vi "HEWH Build String Diagnostics Data.vi"(1 "GEA2":bool, 2 "Pilot (SCFH)":dbl, 5 "ERD Data  2":T6, 9 "ERD Data":string[][](array[string]), 11 "Error In":errorcluster, 12 "Get Gas Data":bool, 13 "Measurement Data":T5, 14 "HEWH Specific DAQ":T1={"HEWH Data"={"HEWH Standard"={"Voltage (Volts)"=-1.0, "Current (Amps)"=-1.0, "Power (Watts)"=-1.0, "WattHours (Wh)"=-1.0, "TC Tree (AVG)"=0.0, "Flow Rate (GPM)"=0.0, "Gallons (Gal)"=0.0, "RTD Out (Deg F)"=0.0, "RTD In (Deg F)"=0.0, "RTD Amb (Deg F)"=0.0, "TC Down"=0.0, "UE Event Lead"=0, "LE Event Lead"=0, "TC Tree Array"=[]}, "PRAT"={"Power (Watts) A"=0.0, "Power (Watts) B"=0.0, "Power (Watts) C"=0.0, "Power (Watts) D"=0.0, "TC1"=0.0, "TC2"=0.0, "TC3"=0.0, "TC4"=0.0, "WattHours (Wh) A"=0.0, "WattHours (Wh) B"=0.0, "WattHours (Wh) C"=0.0, "WattHours (Wh) D"=0.0, "Ambient"=0.0, "Extra Temp"=0.0}, "Additional Power Data"={"Vthd"=0.0, "Frequency (Hz)"=0.0, "Apparent Power (VA)"=0.0, "Power Factor"=0.0, "Current Crest Factor"=0.0, "Voltage Crest Factor"=0.0, "Integration Time (sec)"=0.0}}, "Flow Valve % Open"=0.0, "Power State"={"UE"=FALSE, "LE"=FALSE, "COMP"=FALSE, "FANS"=FALSE}, "Power Analyzer"=enum."APLUS", "Flow Valve uA Output"=0, "Gallons Start (Gal)"=0.0, "PI Output"=0.0}) -> (6 "Power Display":T3, 10 "Appliance Data":string[][](array[string]), 15 "Error Out":errorcluster)   [LabVIEW 2020]
uses:
  Type Definitions/HEWH Power Elements.ctl
  Drivers/GEA3 Toolkit/LabVIEW GEA3 Rev2 API Toolkit LV2016/Water Heating Specific/Type Definitions/GEA3 HEWH ERD Data.ctl
  Drivers/GEA3 Toolkit/LabVIEW GEA3 Rev2 API Toolkit LV2016/Water Heating Specific/Type Definitions/GEA3 HEWH Mixing Valve.ctl
  Drivers/Alicat Gas Meter Driver/Sub-VIs/Data Cluster.ctl
  Type Definitions/HEWH Specific DAQ.ctl
  Type Definitions/HEWH Power Data.ctl
  Utility/Type Definitions/UTILITY Power Analyzer.ctl
panel:
  # "Totalizer Timer"
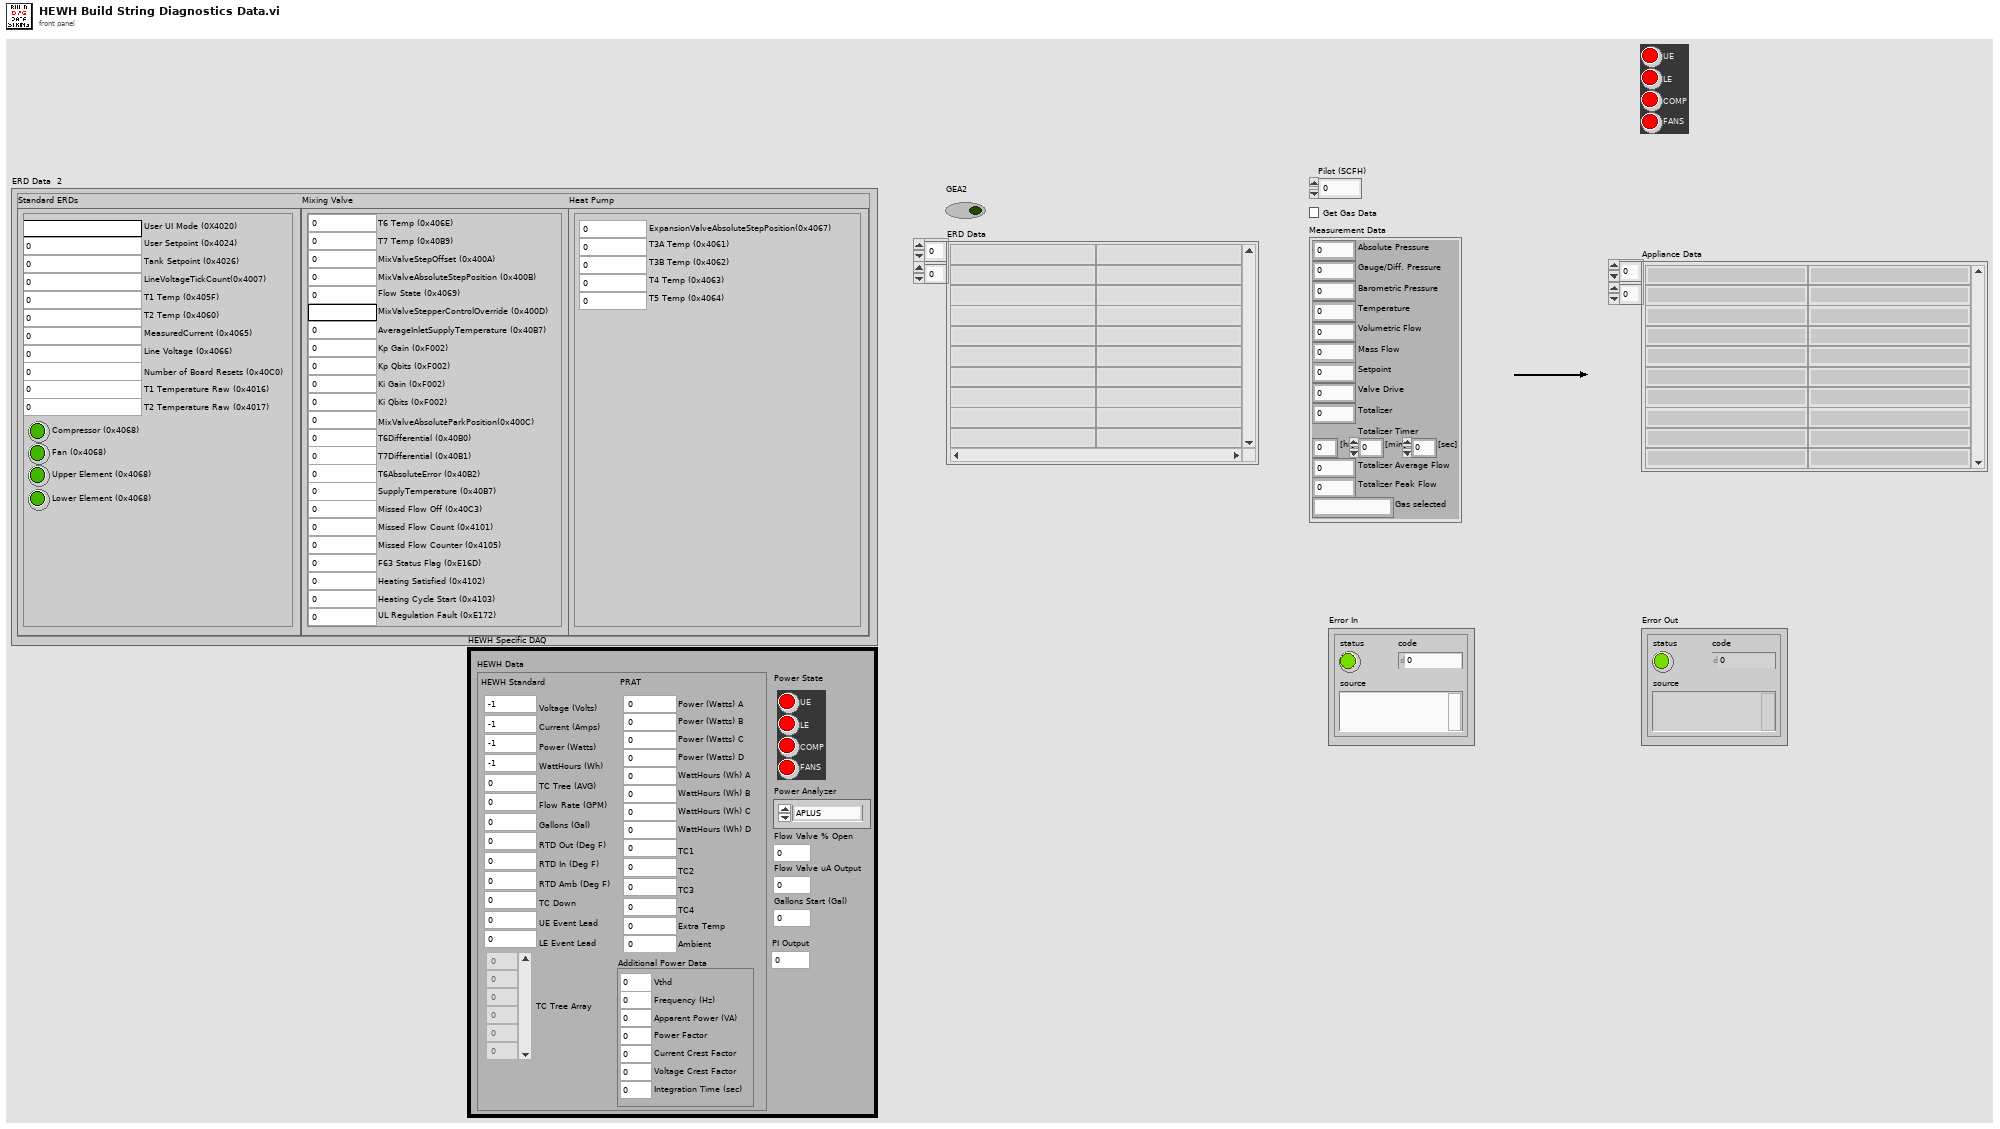
[diagram p1: front panel]
types:
  T1 = typedef "HEWH Specific DAQ.ctl" = cluster{"HEWH Data":T2, "Flow Valve % Open":dbl, "Power State":T3, "Power Analyzer":T4, "Flow Valve uA Output":i32, "Gallons Start (Gal)":dbl, "PI Output":dbl}
  T2 = typedef "HEWH Power Data.ctl" = cluster{"HEWH Standard":cluster{"Voltage (Volts)":dbl, "Current (Amps)":dbl, "Power (Watts)":dbl, "WattHours (Wh)":dbl, "TC Tree (AVG)":dbl, "Flow Rate (GPM)":dbl, "Gallons (Gal)":dbl, "RTD Out (Deg F)":dbl, "RTD In (Deg F)":dbl, "RTD Amb (Deg F)":dbl, "TC Down":dbl, "UE Event Lead":i32, "LE Event Lead":i32, "TC Tree Array":dbl[]}, "PRAT":cluster{"Power (Watts) A":dbl, "Power (Watts) B":dbl, "Power (Watts) C":dbl, "Power (Watts) D":dbl, "TC1":dbl, "TC2":dbl, "TC3":dbl, "TC4":dbl, "WattHours (Wh) A":dbl, "WattHours (Wh) B":dbl, "WattHours (Wh) C":dbl, "WattHours (Wh) D":dbl, "Ambient":dbl, "Extra Temp":dbl}, "Additional Power Data":cluster{"Vthd":dbl, "Frequency (Hz)":dbl, "Apparent Power (VA)":dbl, "Power Factor":dbl, "Current Crest Factor":dbl, "Voltage Crest Factor":dbl, "Integration Time (sec)":dbl}}
  T3 = typedef "HEWH Power Elements.ctl" = cluster{"UE":bool, "LE":bool, "COMP":bool, "FANS":bool}
  T4 = typedef "UTILITY Power Analyzer.ctl" = enum16{"", "APLUS", "WT210", "WT500", "WT300", "OSI", "Debug", "WT230", "WT300_1", "WT300_2"}
  T5 = typedef "Data Cluster.ctl" = cluster{"Absolute Pressure":dbl, "Gauge/Diff. Pressure":dbl, "Barometric Pressure":dbl, "Temperature":dbl, "Volumetric Flow":dbl, "Mass Flow":dbl, "Setpoint":dbl, "Valve Drive":dbl, "Totalizer":dbl, "[hr]":dbl, "[min]":dbl, "[sec]":dbl, "Totalizer Average Flow":dbl, "Totalizer Peak Flow":dbl, "Gas selected":string}
  T6 = typedef "GEA3 HEWH ERD Data.ctl" = cluster{"Mixing Valve":T7, "Standard ERDs":cluster{"User UI Mode (0X4020)":string, "User Setpoint (0x4024)":u16, "Compressor (0x4068)":bool, "Lower Element (0x4068)":bool, "Upper Element (0x4068)":bool, "Fan (0x4068)":bool, "T1 Temp (0x405F)":dbl, "T2 Temp (0x4060)":dbl, "Line Voltage (0x4066)":dbl, "MeasuredCurrent (0x4065)":dbl, "LineVoltageTickCount(0x4007)":u16, "Number of Board Resets (0x40C0)":u16, "T1 Temperature Raw (0x4016)":u16, "T2 Temperature Raw (0x4017)":u16, "Tank Setpoint (0x4026)":u16}, "Heat Pump":cluster{"ExpansionValveAbsoluteStepPosition(0x4067)":i16, "T3A Temp (0x4061)":dbl, "T3B Temp (0x4062)":dbl, "T4 Temp (0x4063)":dbl, "T5 Temp (0x4064)":dbl}}
  T7 = typedef "GEA3 HEWH Mixing Valve.ctl" = cluster{"T7 Temp (0x40B9)":dbl, "MixValveStepOffset (0x400A)":i16, "MixValveAbsoluteStepPosition (0x400B)":i16, "Flow State (0x4069)":u8, "MixValveStepperControlOverride (0x400D)":string, "AverageInletSupplyTemperature (0x40B7)":dbl, "T6 Temp (0x406E)":dbl, "Kp Gain (0xF002)":u16, "Kp Qbits (0xF002)":u16, "Ki Gain (0xF002)":u16, "Ki Qbits (0xF002)":u16, "MixValveAbsoluteParkPosition(0x400C)":i16, "T7Differential (0x40B1)":dbl, "T6Differential (0x40B0)":dbl, "SupplyTemperature (0x40B7)":dbl, "Missed Flow Off (0x40C3)":u8, "T6AbsoluteError (0x40B2)":dbl, "Missed Flow Count (0x4101)":u16, "Missed Flow Counter (0x4105)":u16, "F63 Status Flag (0xE16D)":u16, "Heating Satisfied (0x4102)":u16, "Heating Cycle Start (0x4103)":u16, "UL Regulation Fault (0xE172)":u8}
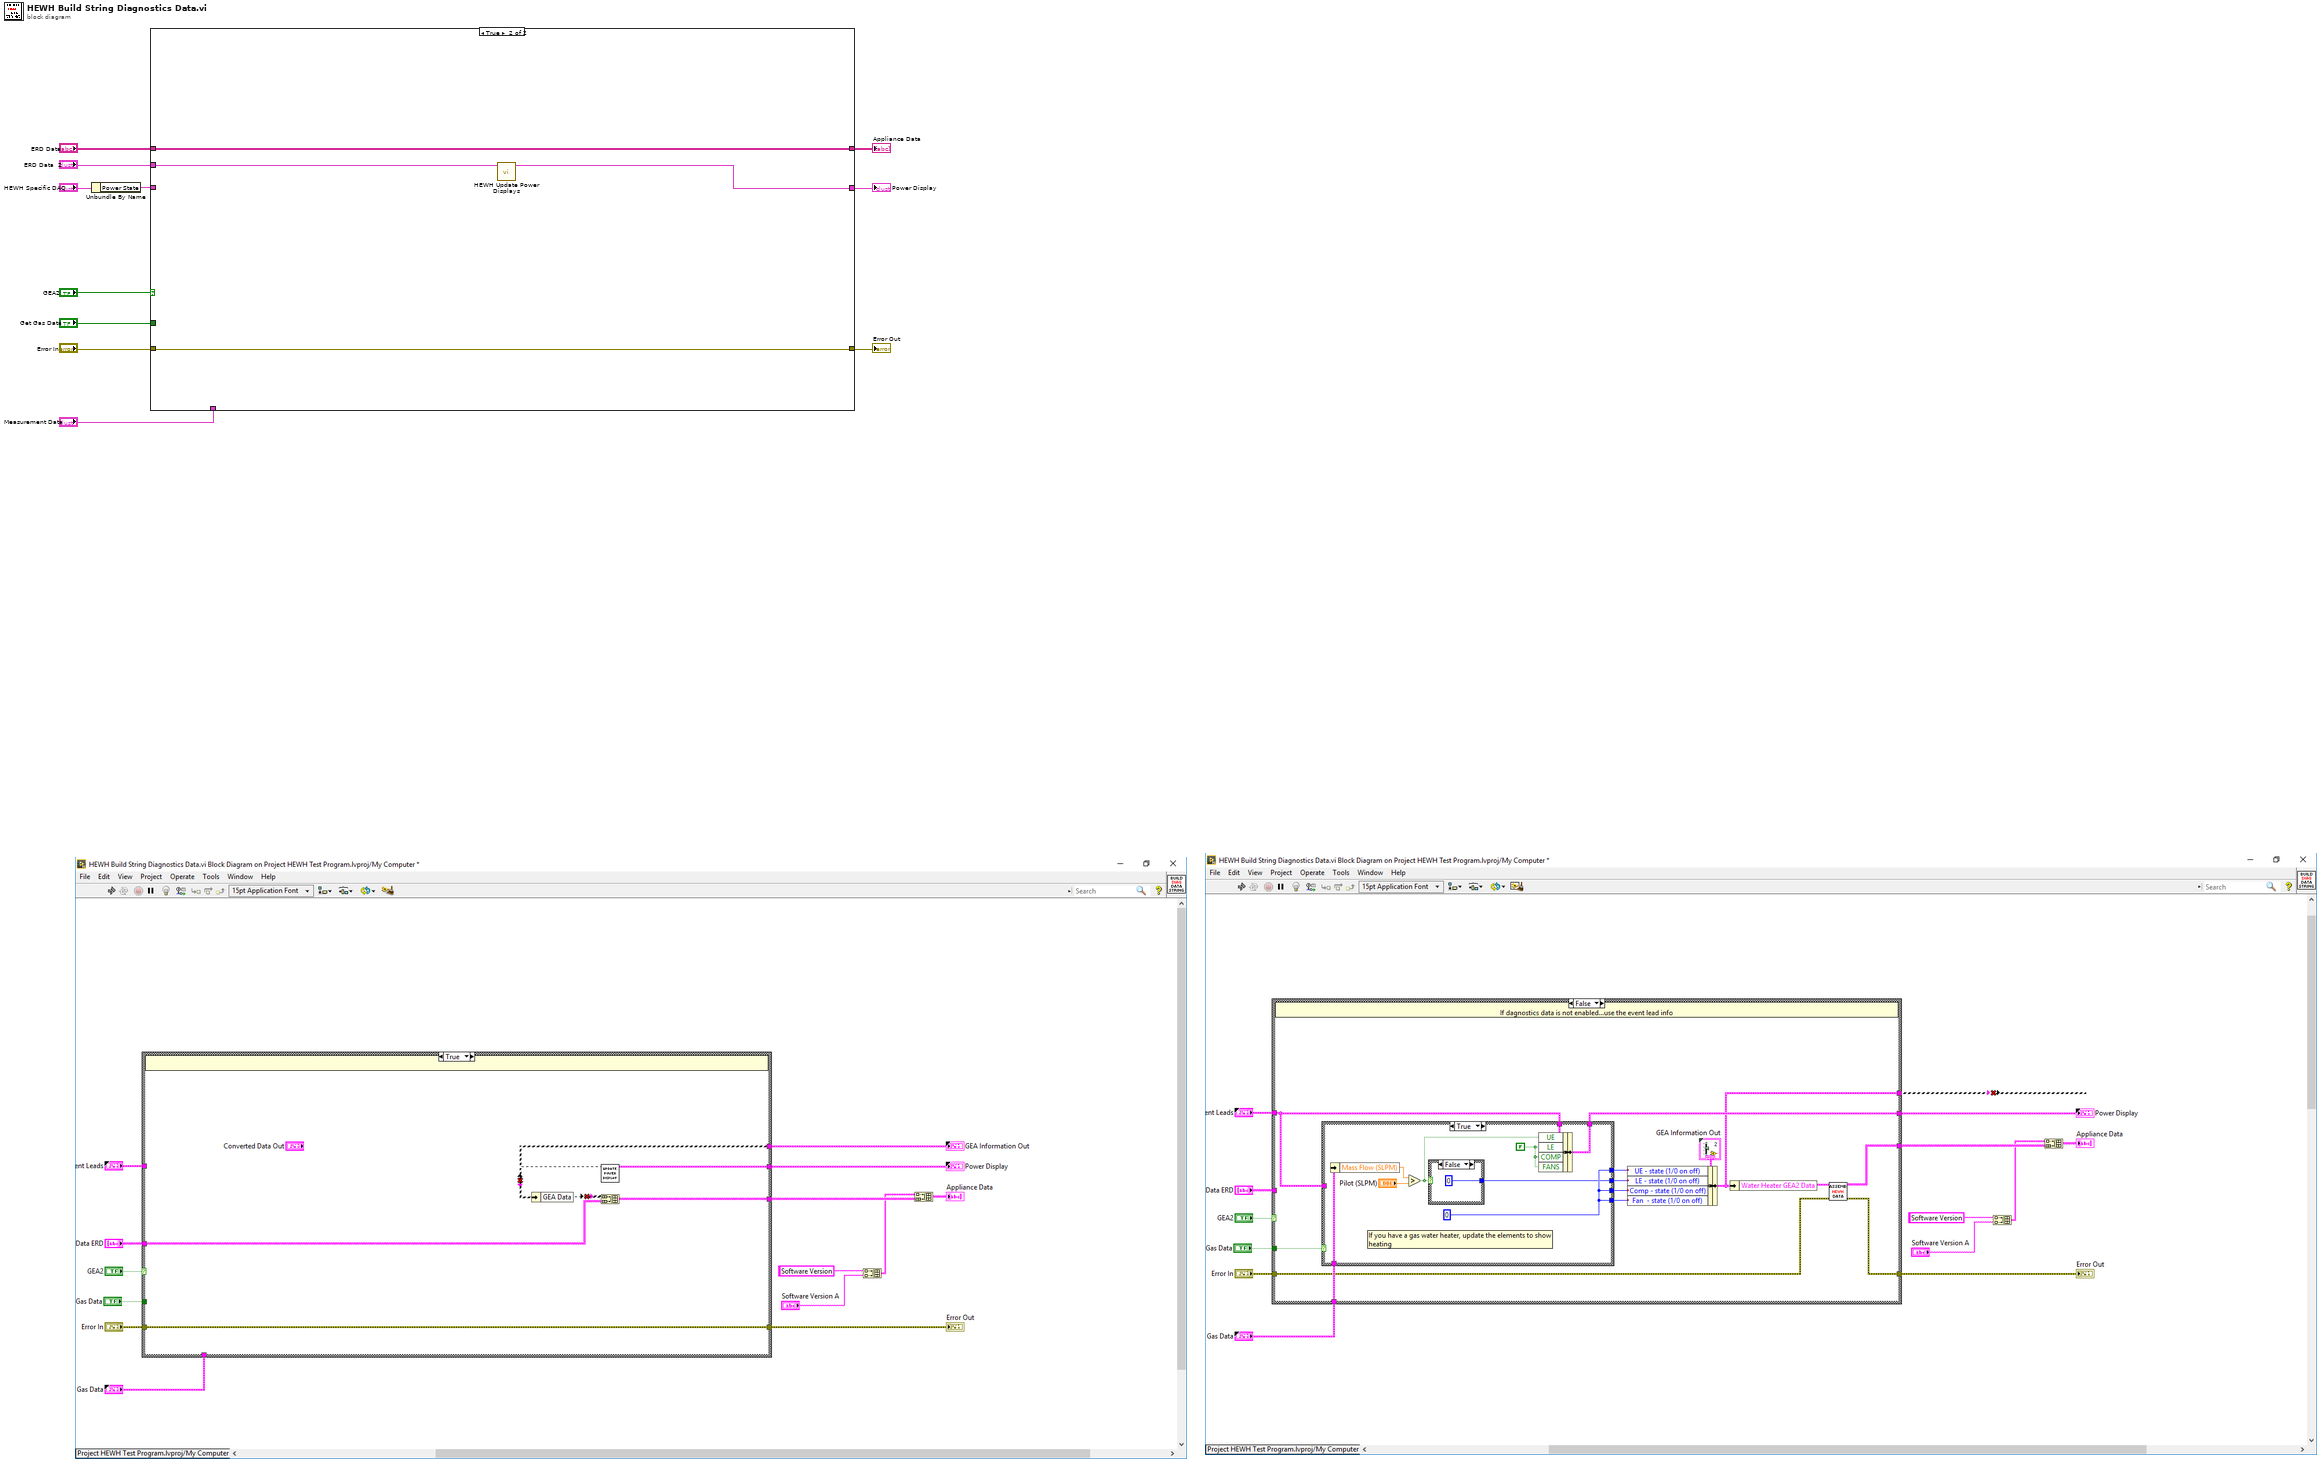
[diagram p0: block diagram]
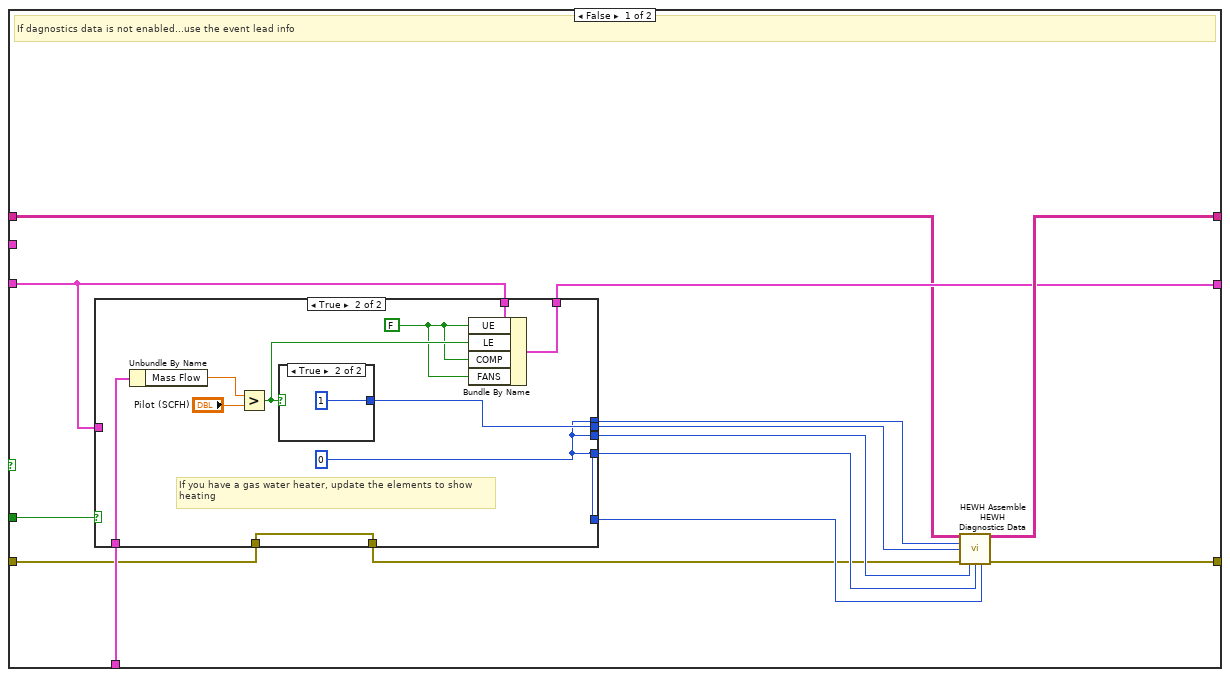
[diagram p2: hidden frame]
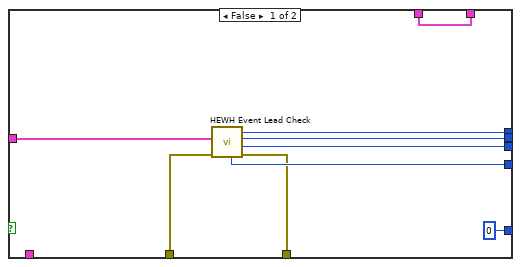
[diagram p3: hidden frame]
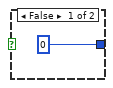
[diagram p4: hidden frame]
diagram:
  n1 = Unbundle By Name("HEWH Specific DAQ") -> ("Power State"=w1:T3)
  n2 = case shown="True" "GEA2" {
    tunnel: [w20 w50] -> w10
    tunnel: w1 -> [w21 _]
    tunnel: "ERD Data" -> [w19 w47]
    tunnel: [w24 w47] -> w4
    tunnel: "Error In" -> [w13 w49]
    tunnel: [w25 w49] -> w7
    tunnel: "Measurement Data" -> [w22 _]
    tunnel: "Get Gas Data" -> [w23 _]
    tunnel: "ERD Data  2" -> [_ w48]
    frame False {
      # "If dagnostics data is not enabled...use the event lead info"
      n3 = case shown="True" w23 {
        tunnel: w21 -> [w34 _]
        tunnel: [w33 w36] -> w18
        tunnel: [w32 w36] -> w15
        tunnel: [w31 w36] -> w16
        tunnel: [w30 w41] -> w17
        tunnel: w22 -> [_ w44]
        tunnel: w21 -> [w29 w40]
        tunnel: [w29 w39] -> w20
        tunnel: [i16 0 w36] -> w14
        tunnel: w13 -> [w27 w35]
        tunnel: [w26 w35] -> w12
        frame False {
          n4 = call "HEWH Event Lead Check.vi"("error in (no error)"=w27, "Power State"=w34) -> ("error out"=w26:errorcluster, "Comp"=w31:i16, "LE"=w30:i16, "UE"=w33:i16, "Fans"=w32:i16)  [unwired: 5 in]
        }
        frame True {
          w37 = FALSE ("UE")
          w36 = i16 0
          # "If you have a gas water heater, update the elements to show\nheating"
          n5 = Unbundle By Name(w44) -> ("Mass Flow"=w43:dbl)
          n6 = Greater?(x=w43, y="Pilot (SCFH)") -> (0:w38:bool)
          n7 = case shown="True" w38 {
            tunnel: [i16 0 i16 1] -> w41
            frame False {
            }
            frame True {
            }
          }
          n8 = Bundle By Name(cluster=w40, "UE"=w37, "LE"=w38, "COMP"=w37, "FANS"=w37) -> (w39:T3)
        }
      }
      n9 = call "HEWH Assemble HEWH Diagnostics Data.vi"("Input Updated Data (No GEA) 2"=w19, "UE"=w18, "LE"=w17, "Error In"=w12, "Comp"=w16, "Fan"=w15, "DLB"=w14) -> ("Output Updated Data (No GEA)"=w24:string[][], "Error Out"=w25:errorcluster)  [unwired: 7 in]
    }
    frame True {
      n10 = call "HEWH Update Power Displays.vi"("ERD Data  2"=w48) -> ("POWER Out"=w50:T3)  [unwired: 9 in, 1 out]
    }
  }
  "Power Display" <- w10
  "Error Out" <- w7
  "Appliance Data" <- w4
